vi "compute_statistics_data_starter.vi"() -> ()   [LabVIEW 2020]
uses:
  StatisticsData.ctl
  Phase.lvclass
  HasoSlopes.lvclass
  WavefrontReconstructionMode.ctl
  Pupil.lvclass
panel:
  out "Wavefront":sgl[][](graph)
  in  "Haso slopes file name":string="Data\\data_phase_computation.has"
  out "error out":errorcluster
  out "Statistics":T1
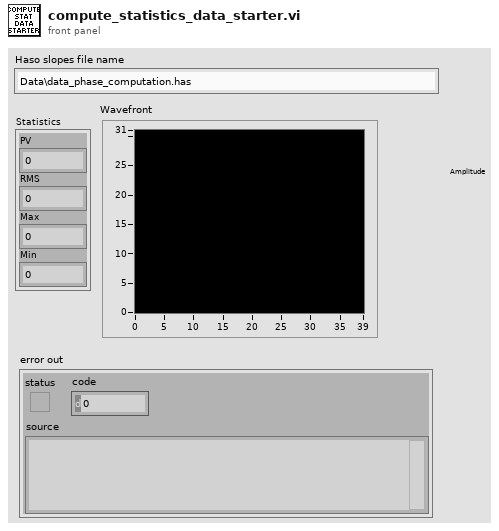
[diagram p1: front panel]
types:
  T1 = typedef "StatisticsData.ctl" = cluster{"PV":sgl, "RMS":dbl, "Max":sgl, "Min":sgl}
  T2 = typedef "WavefrontReconstructionMode.ctl" = enum16{"None", "Modal_Legendre", "Modal_Zernike", "Zonal", "Modal_Zonal_Zernike", "Modal_Zonal_Legendre"}
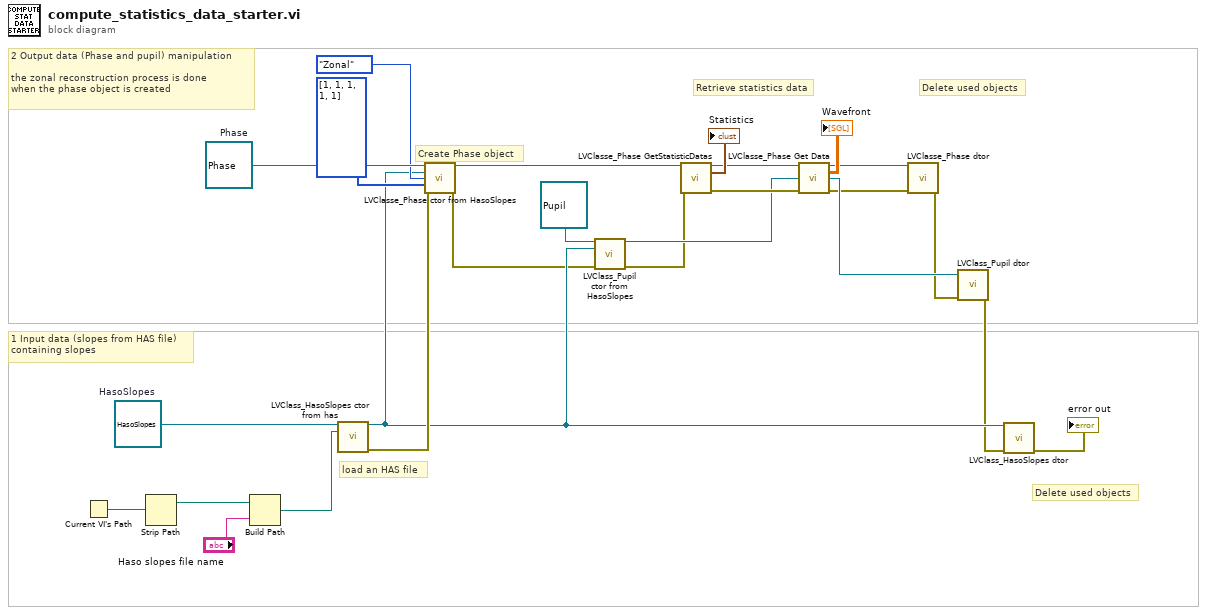
[diagram p0: block diagram]
diagram:
  w20 = refnum<class "HasoSlopes.lvclass"> refnum  # HasoSlopes
  w19 = refnum<class "Phase.lvclass"> refnum  # Phase
  # "Delete used objects"
  # "2 Output data (Phase and pupil) manipulation\n\nthe zonal reconstruction process is done \nwhen the phase object is created"
  # "1 Input data (slopes from HAS file)\ncontaining slopes"
  # "Retrieve statistics data"
  # "Create Phase object"
  # "load an HAS file"
  # "Delete used objects"
  n1 = Current VI's Path() -> (path=w23:path)
  n2 = Strip Path(path=w23) -> (stripped path=w21:path)  [unwired: 1 out]
  n3 = Build Path(base path=w21, name or relative path="Haso slopes file name") -> (appended path=w14:path)
  n4 = call "LVClass_HasoSlopes ctor from has.vi"("HasoSlopes in"=w20, ".has path"=w14) -> ("HasoSlopes out"=w8:refnum<class "HasoSlopes.lvclass">, "error out"=w18:errorcluster)  [unwired: 12 in]
  n5 = call "LVClasse_Phase ctor from HasoSlopes.vi"("Phase in"=w19, "HasoSlopes.lvclass"=w8, "TypePhase"=WavefrontReconstructionMode."Zonal", "Filter"=u8[] [1, 1, 1, 1, 1], "error in (no error)"=w18) -> ("Phase out"=w15:refnum<class "Phase.lvclass">, "error out"=w5:errorcluster)  [unwired: 9 in]
  n6 = call "LVClass_Pupil ctor from HasoSlopes.vi"("Pupil in"=refnum<class "Pupil.lvclass"> refnum, "HasoSlopes.lvclass"=w8, "error in (no error)"=w5) -> ("Pupil out"=w7:refnum<class "Pupil.lvclass">, "error out"=w4:errorcluster)  [unwired: 11 in]
  n7 = call "LVClasse_Phase GetStatisticDatas.vi"("Phase in"=w15, "error in (no error)"=w4) -> ("Phase out"=w12:refnum<class "Phase.lvclass">, "StatisticsData"=→"Statistics":T1, "error out"=w11:errorcluster)  [unwired: 11 in]
  n8 = call "LVClasse_Phase Get Data.vi"("Phase in"=w12, "Pupil"=w7, "error in (no error)"=w11) -> ("Phase out"=w10:refnum<class "Phase.lvclass">, "data"=→"Wavefront":sgl[][], "Pupil (dup)"=w6:refnum<class "Pupil.lvclass">, "error out"=w3:errorcluster)  [unwired: 9 in]
  n9 = call "LVClasse_Phase dtor.vi"("Phase in"=w10, "error in (no error)"=w3) -> ()  [unwired: 12 in, 2 out]
  n10 = call "LVClass_Pupil dtor.vi"("Pupil in"=w6, "error in (no error)"=w3) -> ("error out"=w2:errorcluster)  [unwired: 12 in, 1 out]
  n11 = call "LVClass_HasoSlopes dtor.vi"("HasoSlopes in"=w8, "error in (no error)"=w2) -> ("error out"=→"error out":errorcluster)  [unwired: 12 in, 1 out]
